vi "RTS Point File Subset.vi"(8 "Error In":errorcluster, 10 "Data Input":string[](array[string]), 11 "Point File Input":T1) -> (0 "Error Out":errorcluster, 2 "Next Subset":string[](array[string]), 3 "Point File Output":T1)   [LabVIEW 2018]
uses:
  Type Definitions/RTS Point File.ctl
  <vilib>/Utility/error.llb/whitespace.ctl
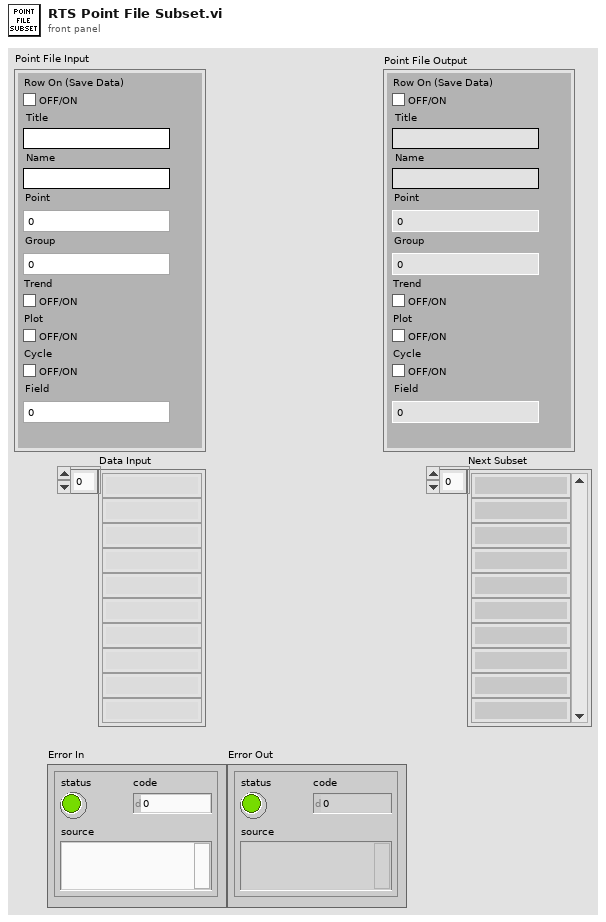
[diagram p1: front panel]
types:
  T1 = typedef "RTS Point File.ctl" = cluster{"Title":string, "Name":string, "Point":u8, "Plot":bool, "Trend":bool, "Cycle":bool, "Field":u8, "Row On (Save Data)":bool, "Group":u8}
  T2 = typedef "whitespace.ctl" = u16
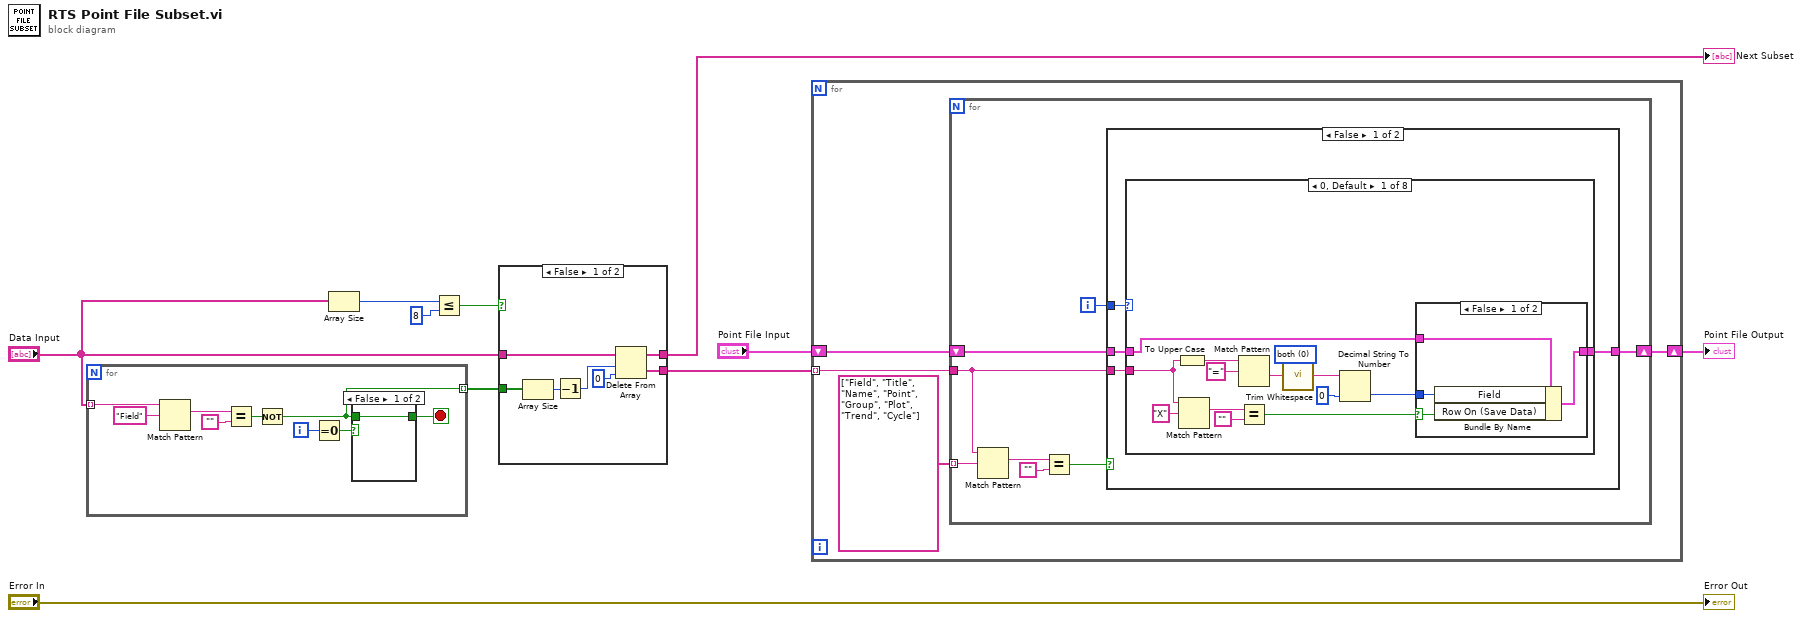
[diagram p0: block diagram]
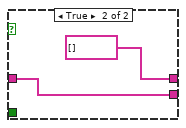
[diagram p2: hidden frame]
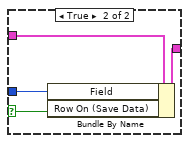
[diagram p3: hidden frame]
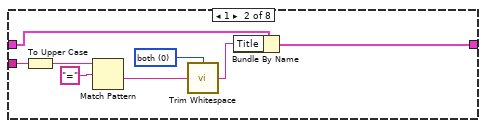
[diagram p4: hidden frame]
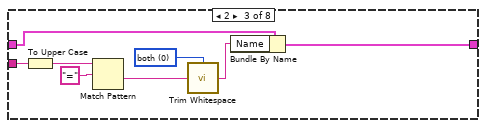
[diagram p5: hidden frame]
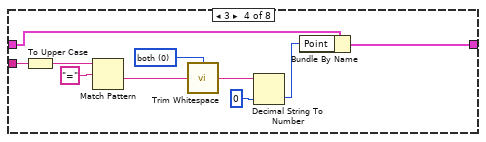
[diagram p6: hidden frame]
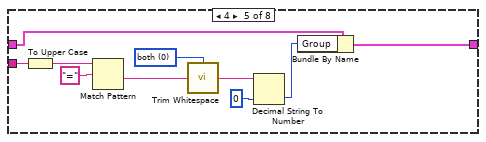
[diagram p7: hidden frame]
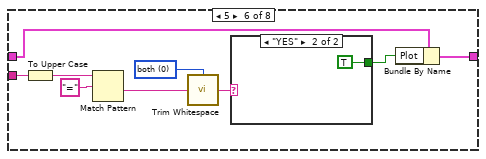
[diagram p8: hidden frame]
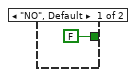
[diagram p9: hidden frame]
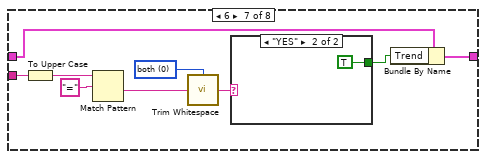
[diagram p10: hidden frame]
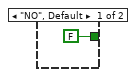
[diagram p11: hidden frame]
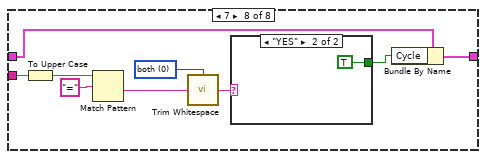
[diagram p12: hidden frame]
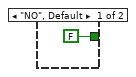
[diagram p13: hidden frame]
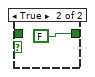
[diagram p15: hidden frame]
diagram:
  n1 = for {
    tunnel: "Data Input" -> [w15] mode=indexing
    tunnel: [w12] -> w7 mode=indexing
    i -> [w14]
    stop <- w11 stop-if-true
    n2 = Match Pattern(string=w15, regular expression="Field") -> (match substring=w18:string)  [unwired: 1 in, 3 out]
    n3 = Equal?(x=w18, y="") -> (x = y?=w16:bool)
    n4 = Not(x=w16) -> (.not. x?=w12:bool)
    n5 = Equal To 0?(x=w14) -> (x = 0?=w13:bool)
    n6 = case shown="False" w13 {
      tunnel: w12 -> [w20 _]
      tunnel: [w20 FALSE] -> w11
      frame False {
      }
      frame True {
      }
    }
  }
  n7 = Array Size(array="Data Input") -> (size(s)=w3:i32)
  n8 = Less Or Equal?(x=w3, y=8) -> (x <= y?=w1:bool)
  n9 = case shown="False" w1 {
    tunnel: [w28 w29] -> w8
    tunnel: w7 -> [w24 _]
    tunnel: [w23 string[] [] ("Data Input")] -> w5
    tunnel: "Data Input" -> [w22 w29]
    frame False {
      n10 = Array Size(array=w24) -> (size(s)=w25:i32)
      n11 = Decrement(x=w25) -> (x-1=w26:i32)
      n12 = Delete From Array(array=w22, length=w26, index=0) -> (deleted portion=w28:string[], array with subset deleted=w23:string[])
    }
    frame True {
    }
  }
  "Next Subset" <- w5
  n13 = for {
    tunnel: w8 -> [w33] mode=indexing
    shift-right: [w34] -> w10
    shift-left: "Point File Input" -> [w32]
    n14 = for {
      tunnel: w33 -> [w38]
      shift-right: [w42] -> w34
      shift-left: w32 -> [w41]
      tunnel: string[] ["Field", "Title", "Name", "Point", "Group", "Plot", "Trend", "Cycle"] ("subarray 2") -> [w40] mode=indexing
      i -> [w39]
      n15 = Match Pattern(string=w38, regular expression=w40) -> (match substring=w37:string)  [unwired: 1 in, 3 out]
      n16 = Equal?(x=w37, y="") -> (x = y?=w35:bool)
      n17 = case shown="False" w35 {
        tunnel: [w46 w138] -> w42
        tunnel: w41 -> [w45 w138]
        tunnel: w39 -> [w44 _]
        tunnel: w38 -> [w43 _]
        frame False {
          n18 = case shown="0, Default" w44 {
            tunnel: [w60 w70 w83 w93 w103 w112 w116 w128] -> w46
            tunnel: w45 -> [w59 w71 w84 w94 w104 w113 w117 w129]
            tunnel: w43 -> [w56 w72 w77 w86 w96 w106 w118 w127]
            frame 0, Default {
              w50 = T2 0 items=["both", "start of string", "end of string"] ("location (both)")
              n19 = To Upper Case(1:w56) -> (0:w52:string)
              n20 = Match Pattern(string=w56, regular expression="X") -> (match substring=w57:string)  [unwired: 1 in, 3 out]
              n21 = Match Pattern(string=w52, regular expression="=") -> (after substring=w49:string)  [unwired: 1 in, 3 out]
              n22 = Equal?(x=w57, y="") -> (x = y?=w47:bool)
              n23 = call <vilib>:"Trim Whitespace.vi"("string"=w49, "location (both)"=w50) -> ("trimmed string"=w48:string)
              n24 = Decimal String To Number(string=w48, default (0L)=u8 0 ("default (0 I32)")) -> (number=w54:u8)  [unwired: 1 in, 1 out]
              n25 = case shown="False" w47 {
                selector: w47 -> [w61 w65]
                tunnel: [w64 w67] -> w60
                tunnel: w59 -> [w63 w68]
                tunnel: w54 -> [w62 w66]
                frame False {
                  n26 = Bundle By Name(cluster=w63, "Field"=w62, "Row On (Save Data)"=w61) -> (w64:T1)
                }
                frame True {
                  n27 = Bundle By Name(cluster=w68, "Field"=w66, "Row On (Save Data)"=w65) -> (w67:T1)
                }
              }
            }
            frame 1 {
              w75 = T2 0 items=["both", "start of string", "end of string"] ("location (both)")
              n28 = To Upper Case(1:w72) -> (0:w73:string)
              n29 = Match Pattern(string=w73, regular expression="=") -> (after substring=w76:string)  [unwired: 1 in, 3 out]
              n30 = call <vilib>:"Trim Whitespace.vi"("string"=w76, "location (both)"=w75) -> ("trimmed string"=w69:string)
              n31 = Bundle By Name(cluster=w71, "Title"=w69) -> (w70:T1)
            }
            frame 2 {
              w80 = T2 0 items=["both", "start of string", "end of string"] ("location (both)")
              n32 = To Upper Case(1:w77) -> (0:w82:string)
              n33 = Match Pattern(string=w82, regular expression="=") -> (after substring=w79:string)  [unwired: 1 in, 3 out]
              n34 = call <vilib>:"Trim Whitespace.vi"("string"=w79, "location (both)"=w80) -> ("trimmed string"=w78:string)
              n35 = Bundle By Name(cluster=w84, "Name"=w78) -> (w83:T1)
            }
            frame 3 {
              w89 = T2 0 items=["both", "start of string", "end of string"] ("location (both)")
              n36 = To Upper Case(1:w86) -> (0:w91:string)
              n37 = Match Pattern(string=w91, regular expression="=") -> (after substring=w88:string)  [unwired: 1 in, 3 out]
              n38 = call <vilib>:"Trim Whitespace.vi"("string"=w88, "location (both)"=w89) -> ("trimmed string"=w87:string)
              n39 = Decimal String To Number(string=w87, default (0L)=u8 0 ("default (0 I32)")) -> (number=w85:u8)  [unwired: 1 in, 1 out]
              n40 = Bundle By Name(cluster=w94, "Point"=w85) -> (w93:T1)
            }
            frame 4 {
              w99 = T2 0 items=["both", "start of string", "end of string"] ("location (both)")
              n41 = To Upper Case(1:w96) -> (0:w101:string)
              n42 = Match Pattern(string=w101, regular expression="=") -> (after substring=w98:string)  [unwired: 1 in, 3 out]
              n43 = call <vilib>:"Trim Whitespace.vi"("string"=w98, "location (both)"=w99) -> ("trimmed string"=w97:string)
              n44 = Decimal String To Number(string=w97, default (0L)=u8 0 ("default (0 I32)")) -> (number=w95:u8)  [unwired: 1 in, 1 out]
              n45 = Bundle By Name(cluster=w104, "Group"=w95) -> (w103:T1)
            }
            frame 5 {
              w110 = T2 0 items=["both", "start of string", "end of string"] ("location (both)")
              n46 = To Upper Case(1:w106) -> (0:w108:string)
              n47 = Match Pattern(string=w108, regular expression="=") -> (after substring=w111:string)  [unwired: 1 in, 3 out]
              n48 = call <vilib>:"Trim Whitespace.vi"("string"=w111, "location (both)"=w110) -> ("trimmed string"=w107:string)
              n49 = case shown="\"YES\"" w107 {
                tunnel: [FALSE TRUE] -> w105
                frame "NO", Default {
                }
                frame "YES" {
                }
              }
              n50 = Bundle By Name(cluster=w113, "Plot"=w105) -> (w112:T1)
            }
            frame 6 {
              w123 = T2 0 items=["both", "start of string", "end of string"] ("location (both)")
              n51 = To Upper Case(1:w118) -> (0:w121:string)
              n52 = Match Pattern(string=w121, regular expression="=") -> (after substring=w124:string)  [unwired: 1 in, 3 out]
              n53 = call <vilib>:"Trim Whitespace.vi"("string"=w124, "location (both)"=w123) -> ("trimmed string"=w120:string)
              n54 = case shown="\"YES\"" w120 {
                tunnel: [FALSE TRUE] -> w119
                frame "NO", Default {
                }
                frame "YES" {
                }
              }
              n55 = Bundle By Name(cluster=w117, "Trend"=w119) -> (w116:T1)
            }
            frame 7 {
              w134 = T2 0 items=["both", "start of string", "end of string"] ("location (both)")
              n56 = To Upper Case(1:w127) -> (0:w132:string)
              n57 = Match Pattern(string=w132, regular expression="=") -> (after substring=w135:string)  [unwired: 1 in, 3 out]
              n58 = call <vilib>:"Trim Whitespace.vi"("string"=w135, "location (both)"=w134) -> ("trimmed string"=w131:string)
              n59 = case shown="\"YES\"" w131 {
                tunnel: [FALSE TRUE] -> w130
                frame "NO", Default {
                }
                frame "YES" {
                }
              }
              n60 = Bundle By Name(cluster=w129, "Cycle"=w130) -> (w128:T1)
            }
          }
        }
        frame True {
        }
      }
    }
  }
  "Point File Output" <- w10
  "Error Out" <- "Error In"
